vi "send_receive(SubVI).vi"(4 "id":i32, 6 "Action":i32, 7 "Data":i32, 8 "error in":errorcluster, 9 "Address":i32, 11 "connection ID":refnum<k5>) -> (0 "error out":errorcluster, 1 "data out":string, 2 "bytes written":i32, 3 "connection ID out":refnum<k5>, 10 "String":string)   [LabVIEW 2009]
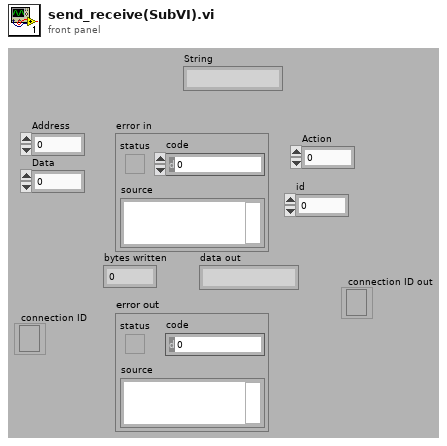
[diagram p1: front panel]
types:
  T1 = enum16{"Standard", "Buffered", "CRLF", "Immediate"}
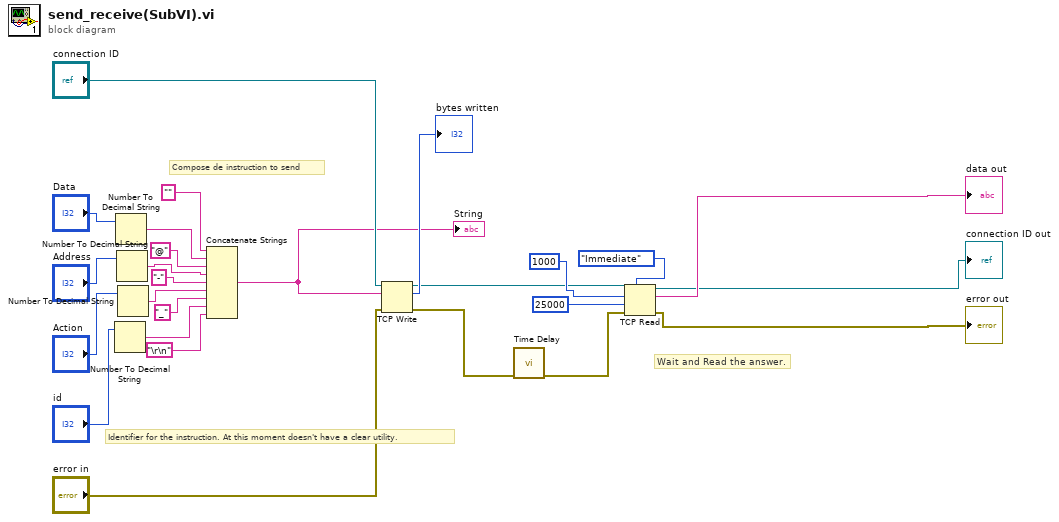
[diagram p0: block diagram]
diagram:
  # "Wait and Read the answer."
  # "Identifier for the instruction. At this moment doesn't have a clear utility."
  # "Compose de instruction to send"
  n1 = Number To Decimal String(number="id") -> (decimal integer string=w13:string)  [unwired: 1 in]
  n2 = Number To Decimal String(number="Data") -> (decimal integer string=w8:string)  [unwired: 1 in]
  n3 = Number To Decimal String(number="Address") -> (decimal integer string=w9:string)  [unwired: 1 in]
  n4 = Number To Decimal String(number="Action") -> (decimal integer string=w10:string)  [unwired: 1 in]
  n5 = Concatenate Strings("", w8, "@" ("string"), w9, "-" ("string"), w10, "_" ("string"), w13, "\r\n") -> (w16:string)
  "String" <- w16
  n6 = TCP Write(connection ID="connection ID", data in=w16, error in (no error)="error in") -> (connection ID out=w4:refnum<k5>, bytes written=→"bytes written":i32, error out=w1:errorcluster)  [unwired: 1 in]
  n7 = call "Time Delay"("error in (no error)"=w1) -> ("error out"=w2:errorcluster)  [unwired: 10 in]
  n8 = TCP Read(connection ID=w4, bytes to read=1000, error in (no error)=w2, 7:T1."Immediate" ("mode (standard)"), 9:25000 ("timeout ms (25000)")) -> (connection ID out=→"connection ID out":refnum<k5>, data out=→"data out":string, error out=→"error out":errorcluster)
